vi "记录生产data.vi"(7 "data输入":string[](array[string]), 11 "写入选项":T1) -> (3 "OK":bool)   [LabVIEW 2017]
uses:
  IOTData.vi
  Sqlite/CBB/UpdateDatas.vi
  Sqlite/CBB/InsertRowData.vi
  Sqlite/SQLite.lvlib
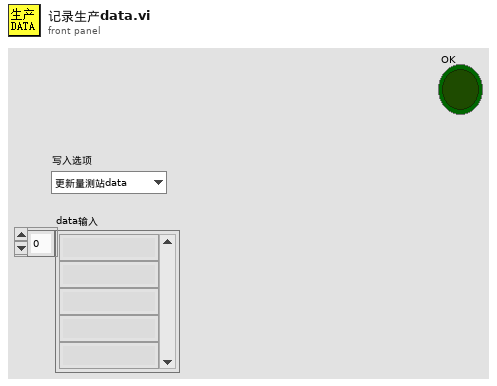
[diagram p1: front panel]
types:
  T1 = typedef "写入选项.ctl" = enum16{"更新量测站data", "更新动子1&2状态", "更新动子3&4状态", "更新量测站CT", "更新动子1&2CT", "更新动子3&4CT", "更新ERData", "更新IOT"}
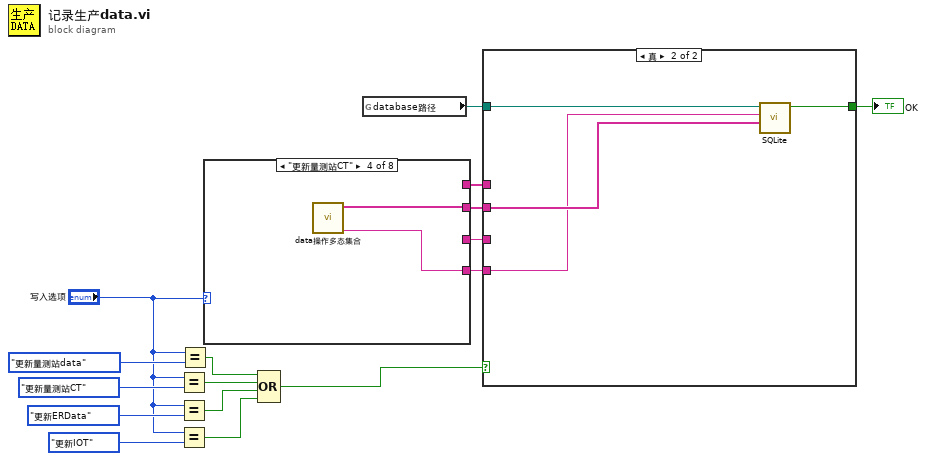
[diagram p0: block diagram]
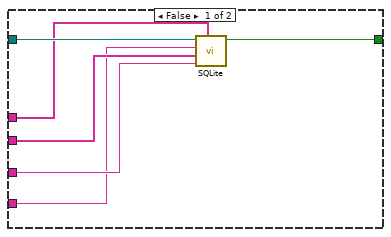
[diagram p2: hidden frame]
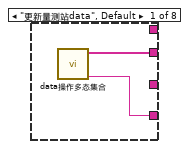
[diagram p3: hidden frame]
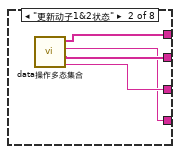
[diagram p4: hidden frame]
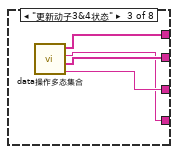
[diagram p5: hidden frame]
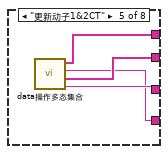
[diagram p6: hidden frame]
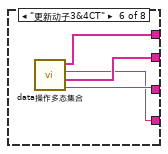
[diagram p7: hidden frame]
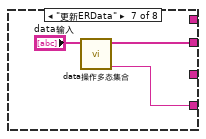
[diagram p8: hidden frame]
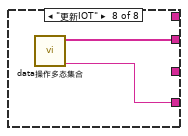
[diagram p9: hidden frame]
diagram:
  n1 = Equal?(x="写入选项", y=写入选项."更新量测站CT") -> (x = y?=w13:bool)
  n2 = Equal?(x="写入选项", y=写入选项."更新ERData") -> (x = y?=w4:bool)
  n3 = Equal?(x="写入选项", y=写入选项."更新IOT") -> (x = y?=w1:bool)
  n4 = Equal?(x="写入选项", y=写入选项."更新量测站data") -> (x = y?=w14:bool)
  n5 = case shown="\"更新量测站CT\"" "写入选项" {
    tunnel: [w18 w22 w25 w28 w31 w35 w38 w41] -> w10
    tunnel: [_ w21 w26 _ w32 w36 _ _] -> w9
    tunnel: [_ w20 w24 _ w30 w34 _ _] -> w8
    tunnel: [w17 w19 w23 w27 w29 w33 w37 w40] -> w6
    frame "更新量测站data", Default {
      n6 = call-poly "data操作多态集合.vi"() -> ("tablename"=w17:string, "data"=w18:string[])  [unwired: 10 in]
    }
    frame "更新动子1&2状态" {
      n7 = call-poly "data操作多态集合.vi"() -> ("Frist ColData"=w20:string, "UpDateData"=w22:string[], "tablename"=w19:string, "UpDateCol"=w21:string[])  [unwired: 8 in]
    }
    frame "更新动子3&4状态" {
      n8 = call-poly "data操作多态集合.vi"() -> ("Frist ColData"=w24:string, "UpDateData"=w25:string[], "tablename"=w23:string, "UpDateCol"=w26:string[])  [unwired: 8 in]
    }
    frame "更新量测站CT" {
      n9 = call-poly "data操作多态集合.vi"() -> ("tablename"=w27:string, "data"=w28:string[])  [unwired: 10 in]
    }
    frame "更新动子1&2CT" {
      n10 = call-poly "data操作多态集合.vi"() -> ("Frist ColData"=w30:string, "UpDateData"=w31:string[], "tablename"=w29:string, "UpDateCol"=w32:string[])  [unwired: 8 in]
    }
    frame "更新动子3&4CT" {
      n11 = call-poly "data操作多态集合.vi"() -> ("Frist ColData"=w34:string, "UpDateData"=w35:string[], "tablename"=w33:string, "UpDateCol"=w36:string[])  [unwired: 8 in]
    }
    frame "更新ERData" {
      n12 = call-poly "data操作多态集合.vi"("data输入"="data输入") -> ("tablename"=w37:string, "data"=w38:string[])  [unwired: 9 in]
    }
    frame "更新IOT" {
      n13 = call-poly "data操作多态集合.vi"() -> ("tablename"=w40:string, "data"=w41:string[])  [unwired: 10 in]
    }
  }
  n14 = Compound Arithmetic op=OR ("复合运算")(w14, w13, w4, w1) -> (w12:bool)
  n15 = global read "数据库全局.vi" "database路径"() -> (w7:path)
  n16 = case shown="真" w12 {
    tunnel: [w47 w51] -> w11
    tunnel: w10 -> [w44 w50]
    tunnel: w7 -> [w46 w49]
    tunnel: w9 -> [w45 _]
    tunnel: w8 -> [w43 _]
    tunnel: w6 -> [w42 w48]
    frame False {
      n17 = call-poly "SQLite.vi"("UpDateCol"=w45, "Frist ColData"=w43, "UpDateData"=w44, "Table Name"=w42, "DbPath"=w46) -> ("OK"=w47:bool)  [unwired: 4 in, 2 out]
    }
    frame True {
      n18 = call-poly "SQLite.vi"("InsertData"=w50, "Table Name"=w48, "DbPath"=w49) -> ("OK"=w51:bool)  [unwired: 6 in, 2 out]
    }
  }
  "OK" <- w11
